vi "target.vi"() -> ()   [LabVIEW 2020]
uses:
  <vilib>/rvi/interface/RandomDataEmulation/niFpgaRandomDataHandleErrors.vi
  matrix_transpose_VIs/32_16_matrix_transpose.vi
  <vilib>/rvi/DataTransferAndStorage/Container/XNode/niFpgaContainer.xnode
  <vilib>/rvi/interface/RandomDataEmulation/nirviRandomDataFpgaReadWriteTemplate.vi
panel:
  out "n":i32
  out "m":i32
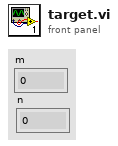
[diagram p1: front panel]
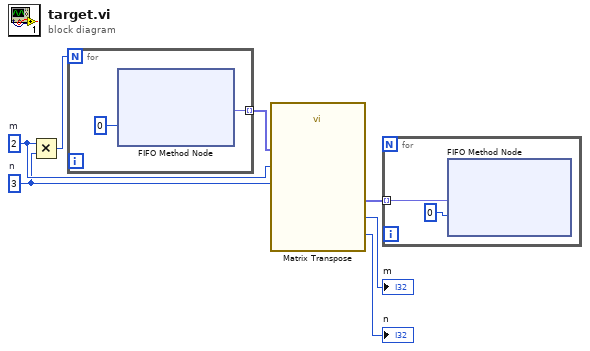
[diagram p0: block diagram]
diagram:
  w4 = 3  # n
  w5 = 2  # m
  n1 = Multiply(x=w5, y=w4) -> (x*y=w7:i32)
  n2 = for {
    N: w7 -> [_]
    tunnel: [w9] -> w6 mode=indexing
    n3 = xnode ("FIFO Method Node")("Timeout"=0) -> ("Element"=w9:fxp<+/-,32,16>)  [unwired: 1 in, 2 out]
  }
  n4 = call-poly "Matrix Transpose.vi"("n"=w4, "m"=w5, "A"=w6) -> ("n"=→"n":i32, "m"=→"m":i32, "B"=w3:fxp<+/-,32,16>[])
  n5 = for {
    tunnel: w3 -> [w10] mode=indexing
    n6 = xnode ("FIFO Method Node")("Element"=w10, "Timeout"=0) -> ()  [unwired: 1 in, 2 out]
  }
